vi "STM_Status_v2.vi"() -> ()   [LabVIEW 2014]
uses:
  <userlib>/Nanonis Prog Interface V5/Nanonis Prog Interface.lvlib
panel:
  in  "dimension size":i32=10000
  out "Current":sgl format="%#_6p"
  out "Tunnelling current":cluster{"Array out":timestamp[], "Array":dbl[]}(graph)
  out "max value STM":dbl=1.6219152410013038e-10
  out "max value prep":dbl=2.1490820234504326e-10
  in  "Emission Current":u16(ring) items=["10", "1", "0.1"]
  out "STM [mBar]":dbl=1.554608664022794e-10 format="%#.2g"
  out "Prep [mBar]":dbl=2.1460036525589032e-10 format="%#.2g"
  out "Pressure":cluster{timestamp[], dbl[]}[](graph)=[{[timestamp(3559596166.680481 s since 1904-01-01), timestamp(3559596187.2546577 s since 1904-01-01)], [1.6219152410013038e-10, 1.5602781566759205e-10]}, {[timestamp(3559596166.680481 s since 1904-01-01), timestamp(3559596187.2546577 s since 1904-01-01)], [2.1490820234504326e-10, 2.1469723221478887e-10]}]
  out "Cryo [K]":dbl=4.220807947684371 format="%#.2g"
  out "STM [K]":dbl=4.597361930995425 format="%#.2g"
  out "Temperature":cluster{timestamp[], dbl[]}[](graph)=[{[timestamp(3559596166.680481 s since 1904-01-01), timestamp(3559596187.2546577 s since 1904-01-01)], [4.221571920530717, 4.221402148787085]}, {[timestamp(3559596166.680481 s since 1904-01-01), timestamp(3559596187.2546577 s since 1904-01-01)], [4.572162263240161, 4.589400389803902]}]
  in  "stop":bool
  in  "refresh [s]":dbl=1.0
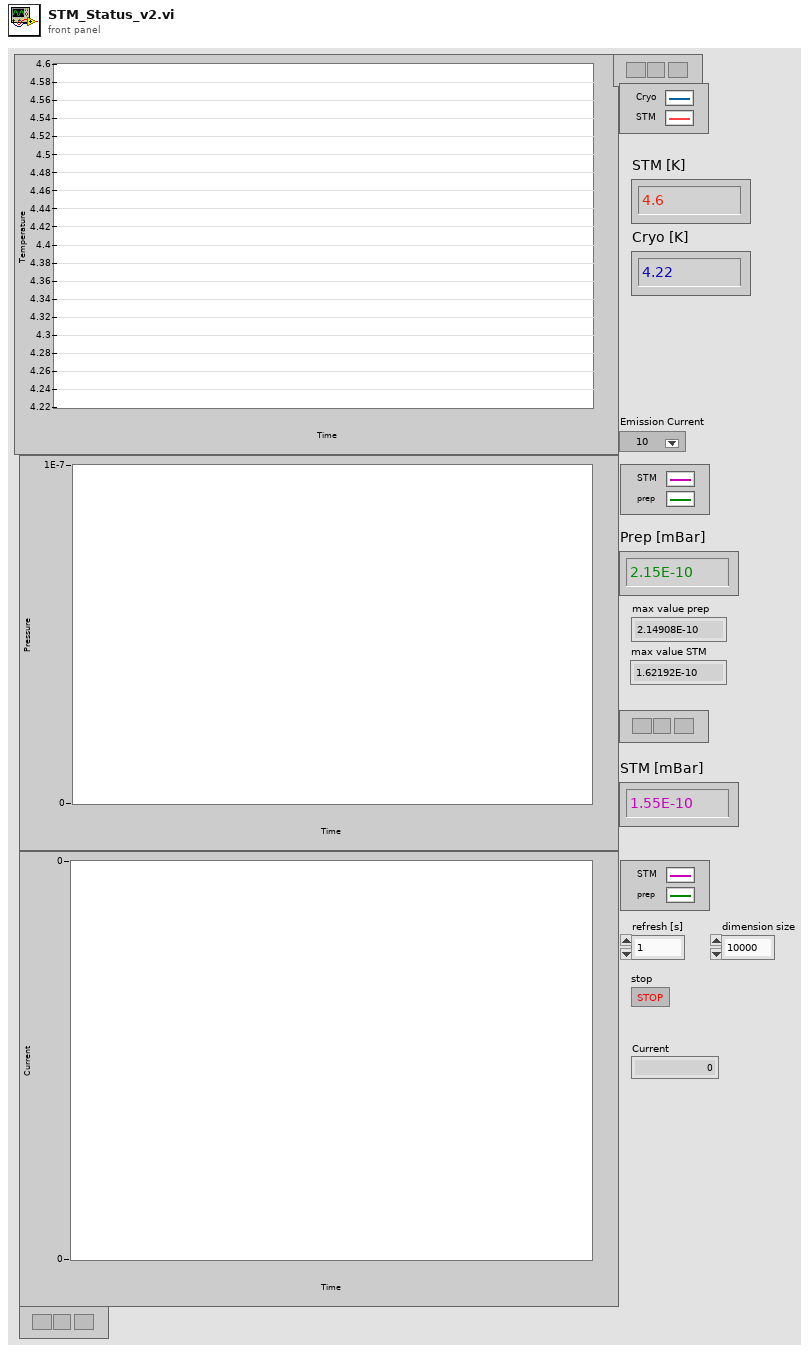
[diagram p1: front panel]
types:
  T1 = cluster{"Array out":timestamp[], "Array":dbl[]}[]
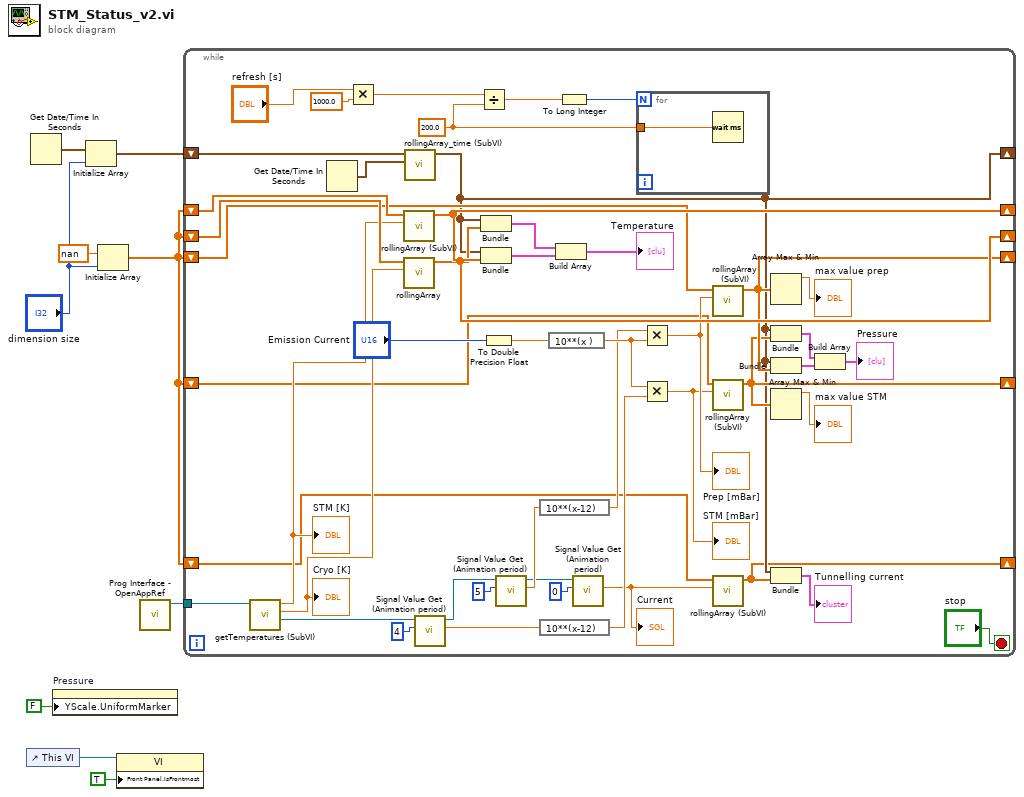
[diagram p0: block diagram]
diagram:
  n1 = control-ref of="This VI"() -> (w8:refnum<vi>)
  n2 = Get Date/Time In Seconds() -> (seconds since 1Jan1904=w3:timestamp)
  n3 = property on="Pressure" class="XYGraph (strict)"("YScale.UniformMarker"=FALSE ("Y Scale.Uniform Marker Spacing?")) -> ()  [unwired: 2 in, 2 out]
  n4 = Initialize Array(w3, "dimension size") -> (w5:timestamp[])
  n5 = Initialize Array(nan ("element"), "dimension size") -> (w2:dbl[])
  n6 = property class="VI"(reference=w8, "Front Panel.IsFrontmost"=TRUE ("Front Panel Window:Is Frontmost")) -> ()  [unwired: 1 in, 2 out]
  n7 = call <userlib>:"Prog Interface - OpenAppRef.vi"() -> ("Application reference"=w9:refnum<vi>)  [unwired: 6 in, 1 out]
  n8 = while {
    tunnel: w9 -> [w52]
    shift-right: [w17] -> _
    shift-left: w5 -> [w55]
    shift-right: [w57] -> _
    shift-left: w2 -> [w54]
    shift-right: [w56] -> _
    shift-left: w2 -> [w53]
    shift-right: [w22] -> _
    shift-left: w2 -> [w23]
    shift-right: [w51] -> _
    shift-left: w2 -> [w50]
    shift-right: [w14] -> _
    shift-left: w2 -> [w18]
    stop <- "stop" stop-if-true
    w11 = 200.0 ("y")
    n9 = call "getTemperatures (SubVI).vi"("Application in"=w52) -> ("Application ref out"=w35:refnum<vi>, "TCryo"=w26:dbl, "TSTM"=w29:dbl)  [unwired: 7 in, 1 out]
    "STM [K]" <- w29
    "Cryo [K]" <- w26
    n10 = Get Date/Time In Seconds() -> (seconds since 1Jan1904=w27:timestamp)
    n11 = Multiply(x="refresh [s]", y=1000.0) -> (x*y=w13:dbl)
    n12 = call "rollingArray (SubVI).vi"("new element/subarray"=w29, "array"=w54) -> ("Array"=w57:dbl[])  [unwired: 9 in]
    n13 = call-poly "rollingArray.vi"("new element/subarray"=w26, "array"=w53) -> ("Array"=w56:dbl[])  [unwired: 9 in]
    n14 = call "rollingArray_time (SubVI).vi"("seconds since 1Jan1904"=w27, "Array in"=w55) -> ("Array out"=w17:timestamp[])  [unwired: 9 in]
    n15 = call <userlib>:"Signal Value Get (Animation period).vi"("Signal index (0-47)"=i8 4, "Application ref in"=w35) -> ("Signal value"=w36:sgl, "Application ref out"=w42:refnum<vi>)  [unwired: 6 in, 1 out]
    n16 = Divide(x=w13, y=w11) -> (x/y=w12:dbl)
    n17 = Bundle("Array out"=w17, "Array"=w56) -> (w45:cluster{"Array out":timestamp[], "Array":dbl[]})  [unwired: 1 in]
    n18 = Bundle("Array out"=w17, "Array"=w57) -> (w44:cluster{"Array out":timestamp[], "Array":dbl[]})  [unwired: 1 in]
    n19 = To Double Precision Float(number="Emission Current") -> (double precision float=w46:dbl)
    n20 = call <userlib>:"Signal Value Get (Animation period).vi"("Signal index (0-47)"=i8 5, "Application ref in"=w42) -> ("Signal value"=w34:sgl, "Application ref out"=w20:refnum<vi>)  [unwired: 6 in, 1 out]
    n21 = expression code="10**(x-12)"(w34) -> (w33:sgl)
    n22 = expression code="10**(x-12)"(w36) -> (w32:sgl)
    n23 = expression code="10**(x )"(w46) -> (w47:dbl)
    n24 = Build Array(w45, w44) -> (→"Temperature":T1)
    n25 = To Long Integer(number=w12) -> (32bit integer=w10:i32)
    n26 = call <userlib>:"Signal Value Get (Animation period).vi"("Signal index (0-47)"=i8 0, "Application ref in"=w20) -> ("Signal value"=w16:sgl)  [unwired: 6 in, 2 out]
    "Current" <- w16
    n27 = for {
      N: w10 -> [_]
      tunnel: w11 -> [w58]
      n28 = Wait (ms)(milliseconds to wait=w58) -> ()  [unwired: 1 out]
    }
    n29 = Multiply(x=w33, y=w47) -> (x*y=w28:dbl)
    "Prep [mBar]" <- w28
    n30 = Multiply(x=w47, y=w32) -> (x*y=w21:dbl)
    "STM [mBar]" <- w21
    n31 = call "rollingArray (SubVI).vi"("new element/subarray"=w28, "array"=w50) -> ("Array"=w51:dbl[])  [unwired: 9 in]
    n32 = call "rollingArray (SubVI).vi"("new element/subarray"=w21, "array"=w23) -> ("Array"=w22:dbl[])  [unwired: 9 in]
    n33 = call "rollingArray (SubVI).vi"("new element/subarray"=w16, "array"=w18) -> ("Array"=w14:dbl[])  [unwired: 9 in]
    n34 = Array Max & Min(array=w51) -> (max value=→"max value prep":dbl)  [unwired: 3 out]
    n35 = Bundle("Array out"=w17, "Array"=w22) -> (w39:cluster{"Array out":timestamp[], "Array":dbl[]})  [unwired: 1 in]
    n36 = Bundle("Array out"=w17, "Array"=w51) -> (w38:cluster{"Array out":timestamp[], "Array":dbl[]})  [unwired: 1 in]
    n37 = Array Max & Min(array=w22) -> (max value=→"max value STM":dbl)  [unwired: 3 out]
    n38 = Bundle("Array out"=w17, "Array"=w14) -> (→"Tunnelling current":cluster{"Array out":timestamp[], "Array":dbl[]})  [unwired: 1 in]
    n39 = Build Array(w39, w38) -> (→"Pressure":T1)
  }
